vi "Determine If Pass.vi"(8 "error in (no error)":errorcluster, 9 "DetermineResult(\"\")":string, 10 "SelectRow(0)":i32, 11 "ExcuseNotesHandler in":refnum<class "ExcuseNotesHandler.lvclass">) -> (0 "error out":errorcluster, 3 "ExcuseNotesHandler out":refnum<class "ExcuseNotesHandler.lvclass">)   [LabVIEW 2015, in "ExcuseNotesHandler.lvclass"]
uses:
  ExcuseNotesHandler.lvclass
  ExcuseNotesHandler.lvclass/ExcuseNotesHandler.ctl
  Global Variable/g_Pos_Determine.vi
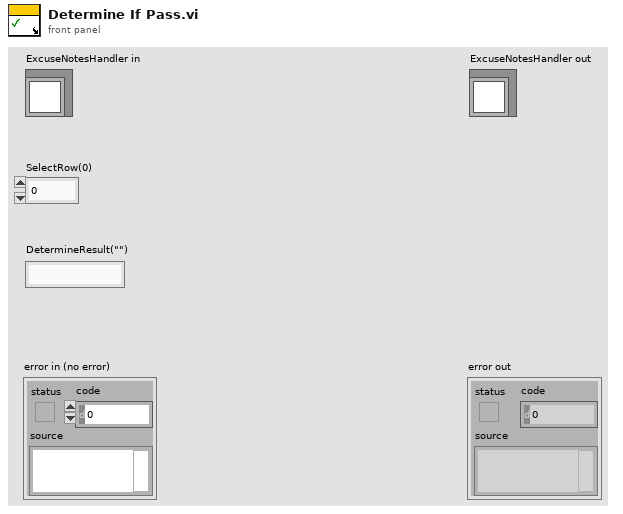
[diagram p1: front panel]
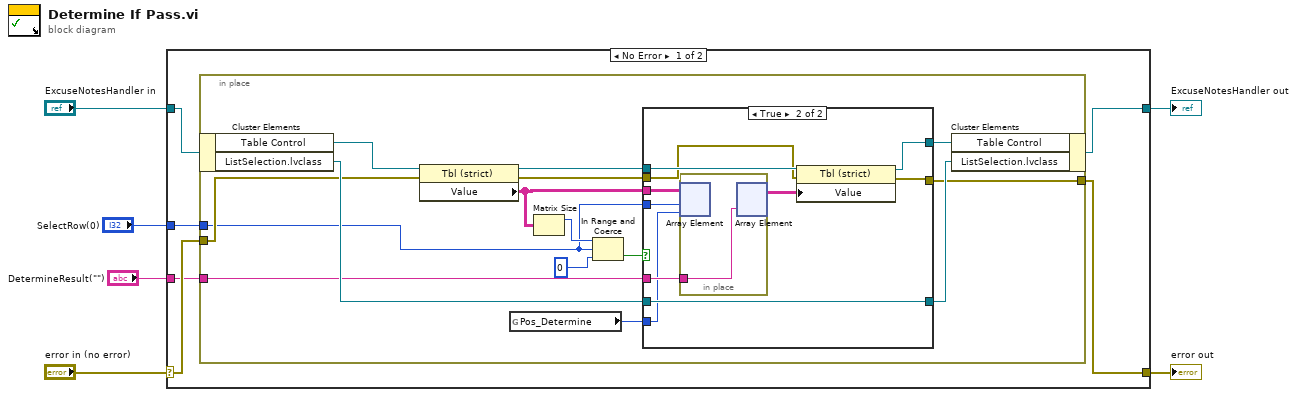
[diagram p0: block diagram]
diagram:
  n1 = case shown="No Error" "error in (no error)" {
    selector: "error in (no error)" -> [w11 w43]
    tunnel: [w9 w43] -> w5
    tunnel: [w10 w42] -> w3
    tunnel: "ExcuseNotesHandler in" -> [w12 w42]
    tunnel: "SelectRow(0)" -> [w8 _]
    tunnel: "DetermineResult(\"\")" -> [w7 _]
    frame No Error {
      n2 = in-place {
        in-place-border: w11 -> [w25]
        in-place-border: [w17] -> w9
        in-place-border: w8 -> [w14]
        in-place-border: w7 -> [w13]
        n3 = in-place-cluster #1(w12) -> ("Table Control"=w27:refnum<vi>, "ListSelection.lvclass"=w26:refnum<class "ListSelection.lvclass">)
        n4 = property class="Tbl (strict)"(reference=w27, error in=w25) -> (reference out=w21:refnum<vi>, error out=w20:errorcluster, "Value"=w22:string[][])
        n5 = global read "g_Pos_Determine.vi" "Pos_Determine"() -> (w15:i32)
        n6 = Matrix Size(0:w22) -> (1:w24:i32)  [unwired: 1 out]
        n7 = In Range and Coerce(upper limit=w24, x=w14, lower limit=0) -> (In Range?=w23:bool)  [unwired: 1 out]
        n8 = case shown="True" w23 {
          tunnel: w22 -> [_ w40]
          tunnel: w21 -> [w30 w37]
          tunnel: w13 -> [_ w38]
          tunnel: w14 -> [_ w39]
          tunnel: w20 -> [w28 w36]
          tunnel: [w30 w34] -> w19
          tunnel: w26 -> [w29 w33]
          tunnel: [w29 w33] -> w18
          tunnel: [w28 w32] -> w17
          tunnel: w15 -> [_ w31]
          frame False {
          }
          frame True {
            n9 = in-place {
              in-place-border: w38 -> [w41]
              n10 = in-place-array #2(w40, w39, w31) -> ()  [unwired: 1 out]
              n11 = in-place-array #2(w41) -> (w35:string[][])  [unwired: 2 out]
            }
            n12 = property class="Tbl (strict)"(reference=w37, error in=w36, "Value"=w35) -> (reference out=w34:refnum<vi>, error out=w32:errorcluster)
          }
        }
        n13 = in-place-cluster #1("Table Control"=w19, "ListSelection.lvclass"=w18) -> (w10:refnum<class "ExcuseNotesHandler.lvclass">)
      }
    }
    frame Error {
    }
  }
  "error out" <- w5
  "ExcuseNotesHandler out" <- w3
